vi "Keithley 2100 Series Read Multiple.vi"() -> ()   [LabVIEW 2020]
doc: "This example shows how to select a function and read multiple measurements."
uses:
  Public/Configure/Configure DC Volts.vi
  Public/Configure/Configure AC Volts.vi
  Public/Configure/Configure DC Current.vi
  Public/Configure/Configure AC Current.vi
  Public/Configure/Configure 2 Wire Resistance.vi
  Public/Configure/Configure 4 Wire Resistance.vi
  Keithley 2100 Series.lvlib
panel:
  out "Measurements":dbl[](array[numeric])
  in  "Timeout (10000 ms)":i32=10000 format="%#.6g"
  in  "Sample Count (1)":i32=1 min=1 max=50000
  in  "Function (0: DC Volts)":u16(ring) items=["DC Volts", "AC Volts", "DC Current", "AC Current", "2-Wire Resistance", "4-Wire Resistance"]
  in  "VISA resource name":refnum<visa-resource-name>="GPIB::16"
  # "This example shows how to select a function, \nuse a bus trigger, and read multiple measurements.\n\nInstructions:\n1. Select a VISA resource name,function,Sample Count\n and appropriate timeout.\n2. Run the VI."
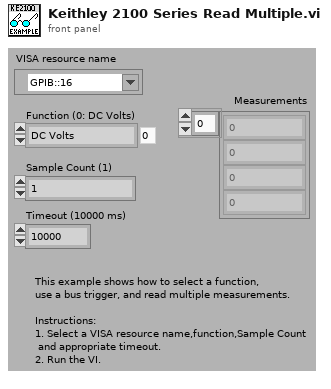
[diagram p1: front panel]
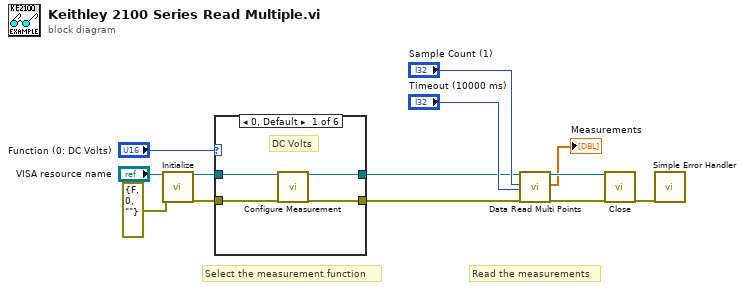
[diagram p0: block diagram]
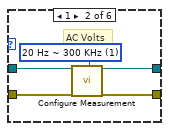
[diagram p2: hidden frame]
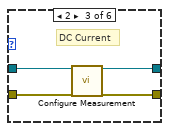
[diagram p3: hidden frame]
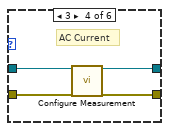
[diagram p4: hidden frame]
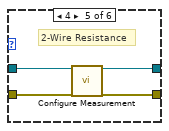
[diagram p5: hidden frame]
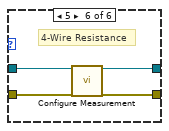
[diagram p6: hidden frame]
diagram:
  # "Read the measurements"
  # "Select the measurement function"
  n1 = call "Initialize.vi"("VISA resource name"="VISA resource name", "error in (no error)"=errorcluster {"status"=FALSE, "code"=0, "source"=""}) -> ("VISA resource name out"=w12:refnum<visa-resource-name>, "error out"=w13:errorcluster)  [unwired: 16 in]
  n2 = case shown="0, Default" "Function (0: DC Volts)" {
    tunnel: w13 -> [w17 w22 w26 w30 w34 w38]
    tunnel: w12 -> [w16 w21 w25 w29 w33 w37]
    tunnel: [w15 w20 w24 w28 w32 w36] -> w1
    tunnel: [w14 w19 w23 w27 w31 w35] -> w2
    frame 0, Default {
      # "DC Volts"
      n3 = call-poly "Configure Measurement.vi"("VISA resource name"=w16, "error in (no error)"=w17) -> ("VISA resource name out"=w14:refnum<visa-resource-name>, "error out"=w15:errorcluster)  [unwired: 16 in]
    }
    frame 1 {
      w18 = u16 1 items=["3 Hz ~ 300 KHz", "20 Hz ~ 300 KHz", "200 Hz ~ 300 KHz"] ("Bandwidth (20 Hz)")
      # "AC Volts"
      n4 = call-poly "Configure Measurement.vi"("VISA resource name"=w21, "error in (no error)"=w22, "Bandwidth (20 Hz)"=w18) -> ("VISA resource name out"=w19:refnum<visa-resource-name>, "error out"=w20:errorcluster)  [unwired: 15 in]
    }
    frame 2 {
      # "DC Current"
      n5 = call-poly "Configure Measurement.vi"("VISA resource name"=w25, "error in (no error)"=w26) -> ("VISA resource name out"=w23:refnum<visa-resource-name>, "error out"=w24:errorcluster)  [unwired: 16 in]
    }
    frame 3 {
      # "AC Current"
      n6 = call-poly "Configure Measurement.vi"("VISA resource name"=w29, "error in (no error)"=w30) -> ("VISA resource name out"=w27:refnum<visa-resource-name>, "error out"=w28:errorcluster)  [unwired: 16 in]
    }
    frame 4 {
      # "2-Wire Resistance"
      n7 = call-poly "Configure Measurement.vi"("VISA resource name"=w33, "error in (no error)"=w34) -> ("VISA resource name out"=w31:refnum<visa-resource-name>, "error out"=w32:errorcluster)  [unwired: 16 in]
    }
    frame 5 {
      # "4-Wire Resistance"
      n8 = call-poly "Configure Measurement.vi"("VISA resource name"=w37, "error in (no error)"=w38) -> ("VISA resource name out"=w35:refnum<visa-resource-name>, "error out"=w36:errorcluster)  [unwired: 16 in]
    }
  }
  n9 = call "Data Read Multi Points.vi"("VISA resource name"=w2, "Sample Count (1)"="Sample Count (1)", "Timeout (10000 ms)"="Timeout (10000 ms)", "error in (no error)"=w1) -> ("VISA resource name out"=w6:refnum<visa-resource-name>, "Measurements"=→"Measurements":dbl[], "error out"=w7:errorcluster)  [unwired: 13 in]
  n10 = call "Close.vi"("VISA resource name"=w6, "error in (no error)"=w7) -> ("error out"=w11:errorcluster)  [unwired: 17 in]
  n11 = call <vilib>:"Simple Error Handler.vi"("error in (no error)"=w11) -> ()  [unwired: 4 in, 5 out]
